vi "Get Next Event.vi"(10 "error in (no error)":errorcluster, 11 "event queue in":string[](array[string])) -> (2 "next event":string, 3 "event queue out":string[](array[string]))   [LabVIEW 2023]
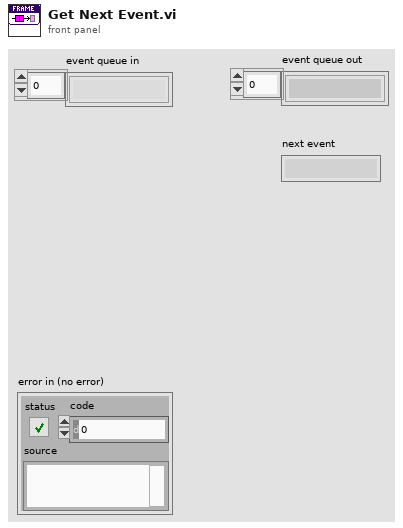
[diagram p1: front panel]
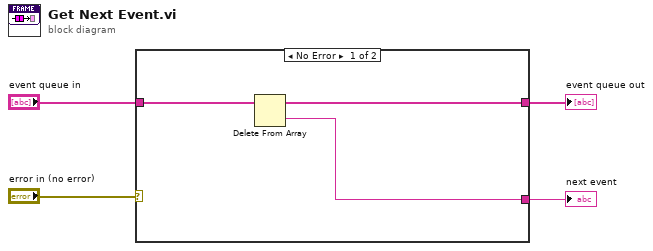
[diagram p0: block diagram]
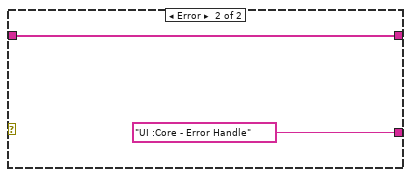
[diagram p2: hidden frame]
diagram:
  n1 = case shown="No Error" "error in (no error)" {
    tunnel: "event queue in" -> [w7 w9]
    tunnel: [w5 "UI :Core - Error Handle" ("Error Handle")] -> w2
    tunnel: [w6 w9] -> w1
    frame No Error {
      n2 = Delete From Array(array=w7) -> (deleted portion=w5:string, array with subset deleted=w6:string[])  [unwired: 2 in]
    }
    frame Error {
    }
  }
  "event queue out" <- w1
  "next event" <- w2
